vi "Calc Type.vi"(11 "Median Calc in":refnum<class "Median Calc.lvclass">) -> (2 "Calc Type":string)   [LabVIEW 2020, in "VolatusCalcs.lvlib" / "Median Calc.lvclass"]
uses:
  Median Calc.lvclass
  Median Calc.lvclass/Median Calc.ctl
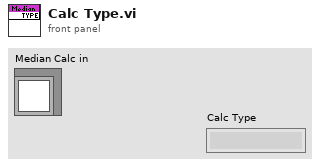
[diagram p1: front panel]
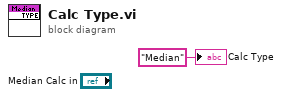
[diagram p0: block diagram]
diagram:
  "Calc Type" <- "Median" ("Calc Type")
